vi "PXI-4130 Main Page Save Action.vi"(8 "error in (no error)":errorcluster, 11 "Device Item Ref in":T1 format="%.0x") -> (0 "error out":errorcluster, 3 "Device Item Ref out":T1 format="%.0x")   [LabVIEW 2009]
uses:
  <vilib>/NI VeriStand/Custom Device API/Custom Device API.lvlib
  <vilib>/NI VeriStand/Custom Device API/Get Item Property (String).vi
  PXI-4130 Global Variable.vi
  PXI-4130 Custom Device.lvlib
  <vilib>/NI VeriStand/Custom Device API/Custom Device Item Ref.ctl
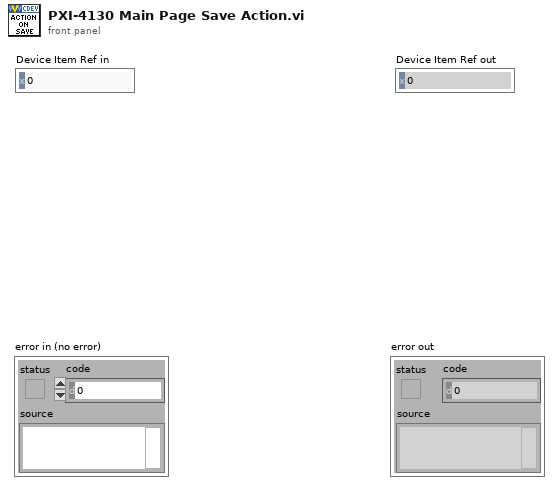
[diagram p1: front panel]
types:
  T1 = typedef "Custom Device API.lvlib/Custom Device Item Ref.ctl" = u64
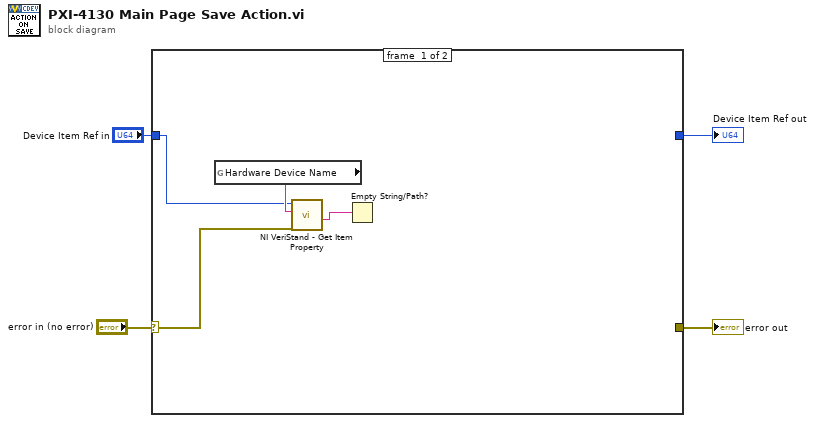
[diagram p0: block diagram]
diagram:
  n1 = case shown="No Error" "error in (no error)" {
    selector: "error in (no error)" -> [w6 w10]
    tunnel: [_ w10] -> w3
    tunnel: "Device Item Ref in" -> [w7 w9]
    tunnel: [_ w9] -> w1
    frame #0 {
      n2 = global read "PXI-4130 Global Variable.vi" "Hardware Device Name"() -> (w8:string)
      n3 = call-poly <vilib>:"NI VeriStand - Get Item Property.vi"("error in (no error)"=w6, "Property Name"=w8, "Item Ref in"=w7) -> ("Value"=w5:string)  [unwired: 5 in, 3 out]
      n4 = Empty String/Path?(string/path=w5) -> ()  [unwired: 1 out]
    }
    frame #1 {
    }
  }
  "error out" <- w3
  "Device Item Ref out" <- w1
